vi "boonton_interface.vi"(6 "error in (no error)":errorcluster, 8 "Command Array":string[](array[string]), 9 "VISA In":refnum<visa-resource-name>) -> (0 "error out":errorcluster, 1 "Command Num.":dbl, 2 "Results":string[](array[string]), 3 "VISA Out":refnum<visa-resource-name>)   [LabVIEW 2011]
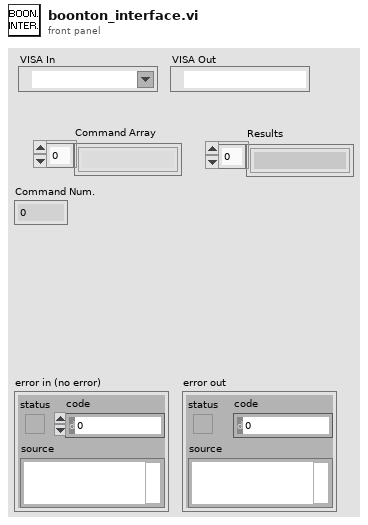
[diagram p1: front panel]
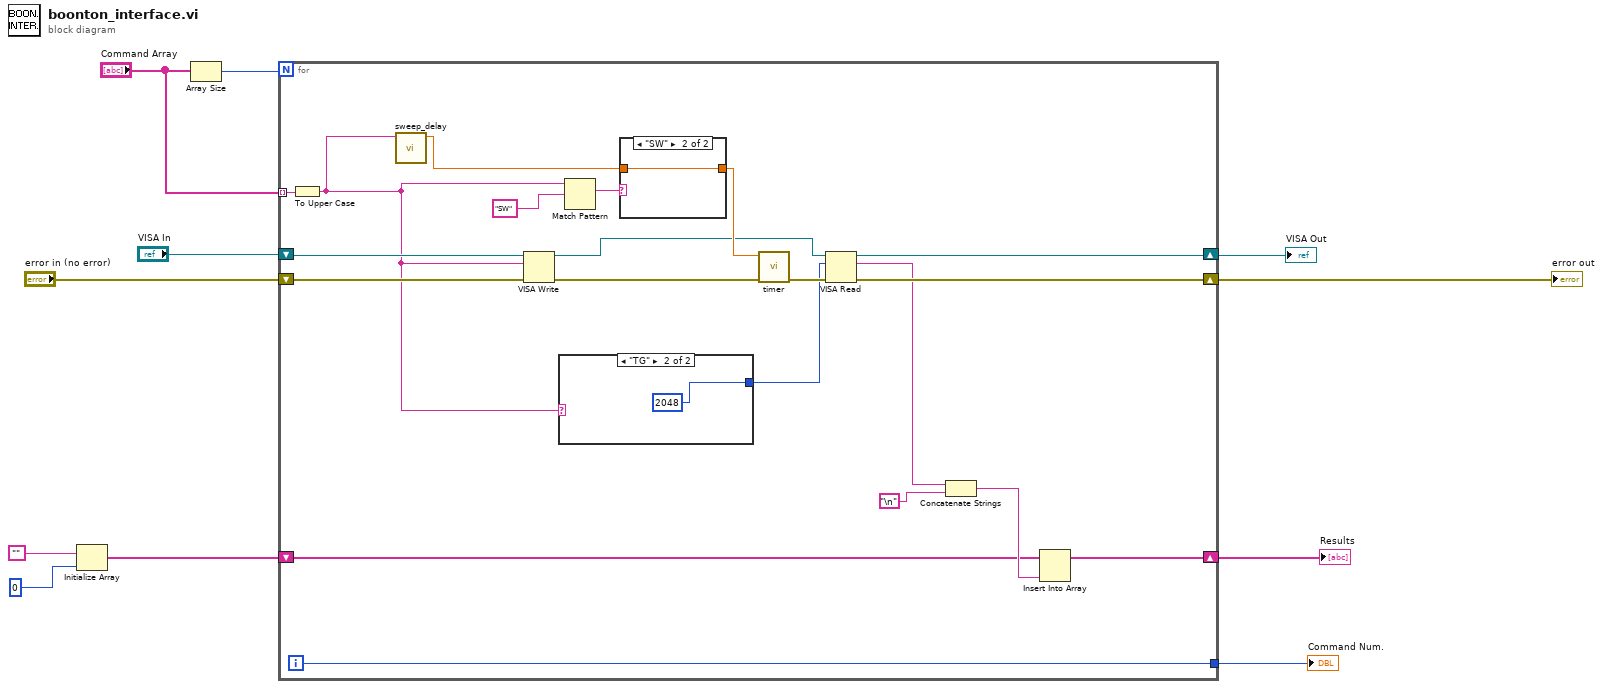
[diagram p0: block diagram]
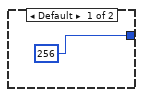
[diagram p2: hidden frame]
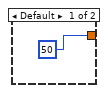
[diagram p3: hidden frame]
diagram:
  n1 = Initialize Array("", 0) -> (w3:string[])
  n2 = Array Size(array="Command Array") -> (size(s)=w11:i32)
  n3 = for {
    N: w11 -> [_]
    tunnel: "Command Array" -> [w31] mode=indexing
    shift-right: [w22] -> w6
    shift-left: "VISA In" -> [w29]
    shift-right: [w20] -> w9
    shift-left: "error in (no error)" -> [w30]
    shift-right: [w13] -> w2
    shift-left: w3 -> [w14]
    tunnel: [w12] -> w1
    i -> [w12]
    n4 = To Upper Case(1:w31) -> (0:w19:string)
    n5 = call "sweep_delay.vi"("Command"=w19) -> ("Delay Time"=w28:dbl)  [unwired: 10 in]
    n6 = VISA Write(VISA resource name=w29, write buffer=w19, error in (no error)=w30) -> (VISA resource name out=w21:refnum<visa-resource-name>, error out=w27:errorcluster)  [unwired: 1 out]
    n7 = case shown="\"TG\"" w19 {
      tunnel: [256 2048] -> w18
      frame Default {
      }
      frame "TG" {
      }
    }
    n8 = Match Pattern(string=w19, regular expression="SW") -> (match substring=w25:string)  [unwired: 1 in, 3 out]
    n9 = case shown="\"SW\"" w25 {
      tunnel: w28 -> [_ w35]
      tunnel: [50 w35] -> w26
      frame Default {
      }
      frame "SW" {
      }
    }
    n10 = call "timer.vi"("error in (no error)"=w27, "Delay Time"=w26) -> ("error out"=w23:errorcluster)  [unwired: 9 in]
    n11 = VISA Read(VISA resource name=w21, byte count=w18, error in (no error)=w23) -> (VISA resource name out=w22:refnum<visa-resource-name>, read buffer=w17:string, error out=w20:errorcluster)  [unwired: 1 out]
    n12 = Concatenate Strings(w17, "\n") -> (w15:string)
    n13 = Insert Into Array(array=w14, new element=w15) -> (w13:string[])  [unwired: 1 in]
  }
  "error out" <- w9
  "VISA Out" <- w6
  "Results" <- w2
  "Command Num." <- w1
